vi "Error - Log.vi"(8 "error in (no error)":errorcluster, 11 "Error Message":T1) -> (0 "error out":errorcluster)   [LabVIEW 2017]
doc: "Maintains a log file which can be checked by personnel.\n[Covers: EH2]"
uses:
  Controls/Error Message.ctl
  Controls/Error Level.ctl
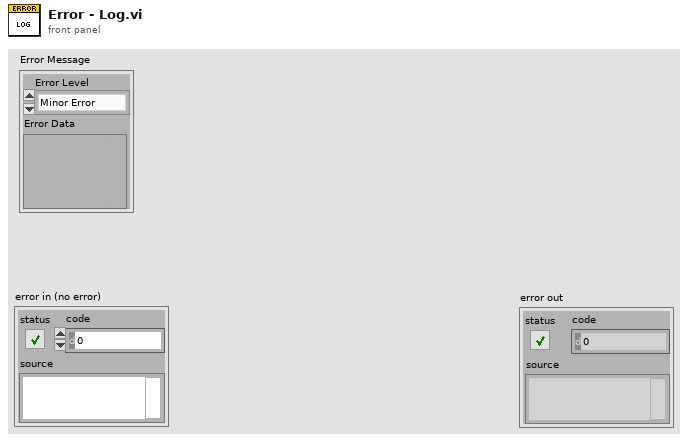
[diagram p1: front panel]
types:
  T1 = typedef "Error Message.ctl" = cluster{"Error Level":T2, "Error Data":variant}
  T2 = typedef "Error Level.ctl" = enum16{"Minor Error", "Wash Cycle Error", "System Error"}
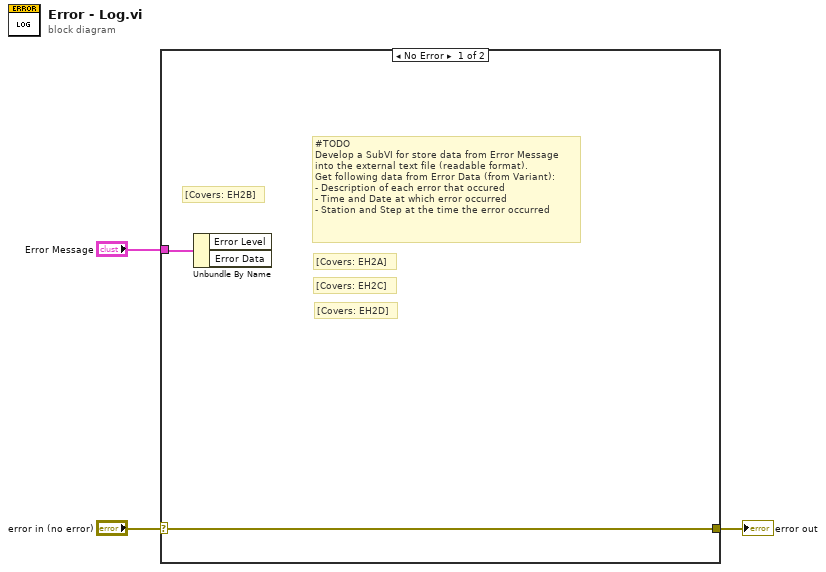
[diagram p0: block diagram]
diagram:
  n1 = case shown="No Error" "error in (no error)" {
    selector: "error in (no error)" -> [w5 w6]
    tunnel: [w5 w6] -> w2
    tunnel: "Error Message" -> [w4 _]
    frame No Error {
      # "[Covers: EH2D]"
      # "[Covers: EH2C]"
      # "[Covers: EH2A]"
      # "[Covers: EH2B]"
      # "#TODO\nDevelop a SubVI for store data from Error Message\ninto the external text file (readable format).\nGet following data from Error Data (from Variant):\n- Description of each error that occured\n- Time and Date at which error occurred\n- Station and Step at the time the error occurred"
      n2 = Unbundle By Name(w4) -> ()  [unwired: 2 out]
    }
    frame Error {
    }
  }
  "error out" <- w2
